vi "UFO_shadow.vi"(11 "Command Queue":refnum<queue>) -> ()   [LabVIEW 2019]
doc: "Window to be displayed below the main UFO window, simulating a shadow. It's opacity should be set to 127."
uses:
  Slave Window Command Message.ctl
  Slave Window Command.ctl
  <vilib>/Utility/miscctls.llb/LVRectTypeDef.ctl
  _Window/Window.lvlib
panel:
  out "UFO Shadow":u16(ring)
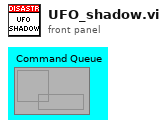
[diagram p1: front panel]
types:
  T1 = enum32{"Invalid", "Standard", "Closed", "Hidden", "Minimized", "Maximized"}
  T2 = typedef "LVRectTypeDef.ctl" = cluster{"Left":i16, "Top":i16, "Right":i16, "Bottom":i16}
  T3 = typedef "Slave Window Command Message.ctl" = cluster{"Command":T4, "Data":variant}
  T4 = typedef "Slave Window Command.ctl" = enum16{"Open", "Set Bounds", "Set Opacity", "Close", "Frame"}
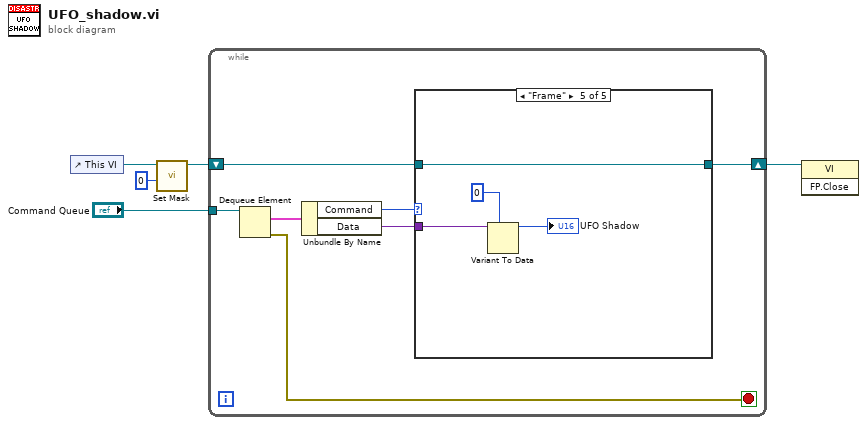
[diagram p0: block diagram]
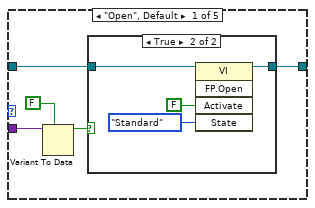
[diagram p2: hidden frame]
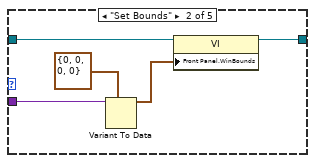
[diagram p4: hidden frame]
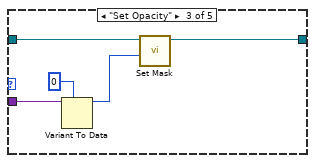
[diagram p5: hidden frame]
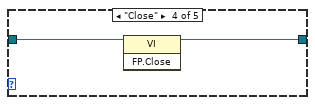
[diagram p6: hidden frame]
diagram:
  n1 = control-ref of="This VI"() -> (w4:refnum<vi>)
  n2 = call "Set Mask.vi"("Alpha (255)"=0, "VI Ref In"=w4) -> ("VI Ref Out"=w3:refnum<vi>)  [unwired: 8 in, 1 out]
  n3 = while {
    tunnel: "Command Queue" -> [w12]
    shift-right: [w6] -> w1
    shift-left: w3 -> [w8]
    stop <- w11 stop-if-true
    n4 = Dequeue Element(queue=w12) -> (element=w10:T3, error out=w11:errorcluster)  [unwired: 2 in, 2 out]
    n5 = Unbundle By Name(w10) -> ("Command"=w9:T4, "Data"=w7:variant)
    n6 = case shown="\"Frame\"" w9 {
      tunnel: w8 -> [w14 w27 w32 w34 w35]
      tunnel: w7 -> [w17 w26 w31 _ w38]
      tunnel: [w13 w23 w28 w33 w35] -> w6
      frame "Open", Default {
        n7 = Variant To Data(type=FALSE, Variant=w17) -> (data=w15:bool)  [unwired: 1 in, 1 out]
        n8 = case shown="True" w15 {
          tunnel: w14 -> [w18 w20]
          tunnel: [w18 w19] -> w13
          frame False {
          }
          frame True {
            n9 = invoke class="VI" method="FP.Open"(reference=w20, "Activate"=FALSE ("Activate?"), "State"=T1."Standard") -> (reference out=w19:refnum<vi>)  [unwired: 2 in, 4 out]
          }
        }
      }
      frame "Set Bounds" {
        n10 = Variant To Data(type=T2 {"Left"=0, "Top"=0, "Right"=0, "Bottom"=0} ("Front Panel Window:Window Bounds"), Variant=w26) -> (data=w24:T2)  [unwired: 1 in, 1 out]
        n11 = property class="VI"(reference=w27, "Front Panel.WinBounds"=w24) -> (reference out=w23:refnum<vi>)  [unwired: 1 in, 1 out]
      }
      frame "Set Opacity" {
        n12 = Variant To Data(type=0 ("Alpha (255)"), Variant=w31) -> (data=w29:i32)  [unwired: 1 in, 1 out]
        n13 = call "Set Mask.vi"("Alpha (255)"=w29, "VI Ref In"=w32) -> ("VI Ref Out"=w28:refnum<vi>)  [unwired: 8 in, 1 out]
      }
      frame "Close" {
        n14 = invoke class="VI" method="FP.Close"(reference=w34) -> (reference out=w33:refnum<vi>)  [unwired: 2 in, 2 out]
      }
      frame "Frame" {
        n15 = Variant To Data(type=u16 0, Variant=w38) -> (data=→"UFO Shadow":u16)  [unwired: 1 in, 1 out]
      }
    }
  }
  n16 = invoke class="VI" method="FP.Close"(reference=w1) -> ()  [unwired: 2 in, 3 out]
